vi "readRawFile.vi"() -> ()   [LabVIEW 2017]
uses:
  <vilib>/vision/NI_Vision_Development_Module.lvlib
panel:
  out "Histogram Report 2":T1 {"Standard  Variation" format="%.2f"; "Mean Value" format="%.2f"; "Interval Width" format="%.2f"; "Starting Value" format="%.2f"; "Maximal Value" format="%.2f"; "Minimal Value" format="%.2f"}
  out "Histogram Report":T1 {"Standard  Variation" format="%.2f"; "Mean Value" format="%.2f"; "Interval Width" format="%.2f"; "Starting Value" format="%.2f"; "Maximal Value" format="%.2f"; "Minimal Value" format="%.2f"}
  out "Error out":errorcluster
  in  "Raw File Path":path=path "F:/BonTechWrapperLibrary/BonTechWrapperLibrary/x64/Release/test.raw"
  in  "Length":i32=256
  in  "Frame Header":bool
  out "Image":T2(plugin-control)
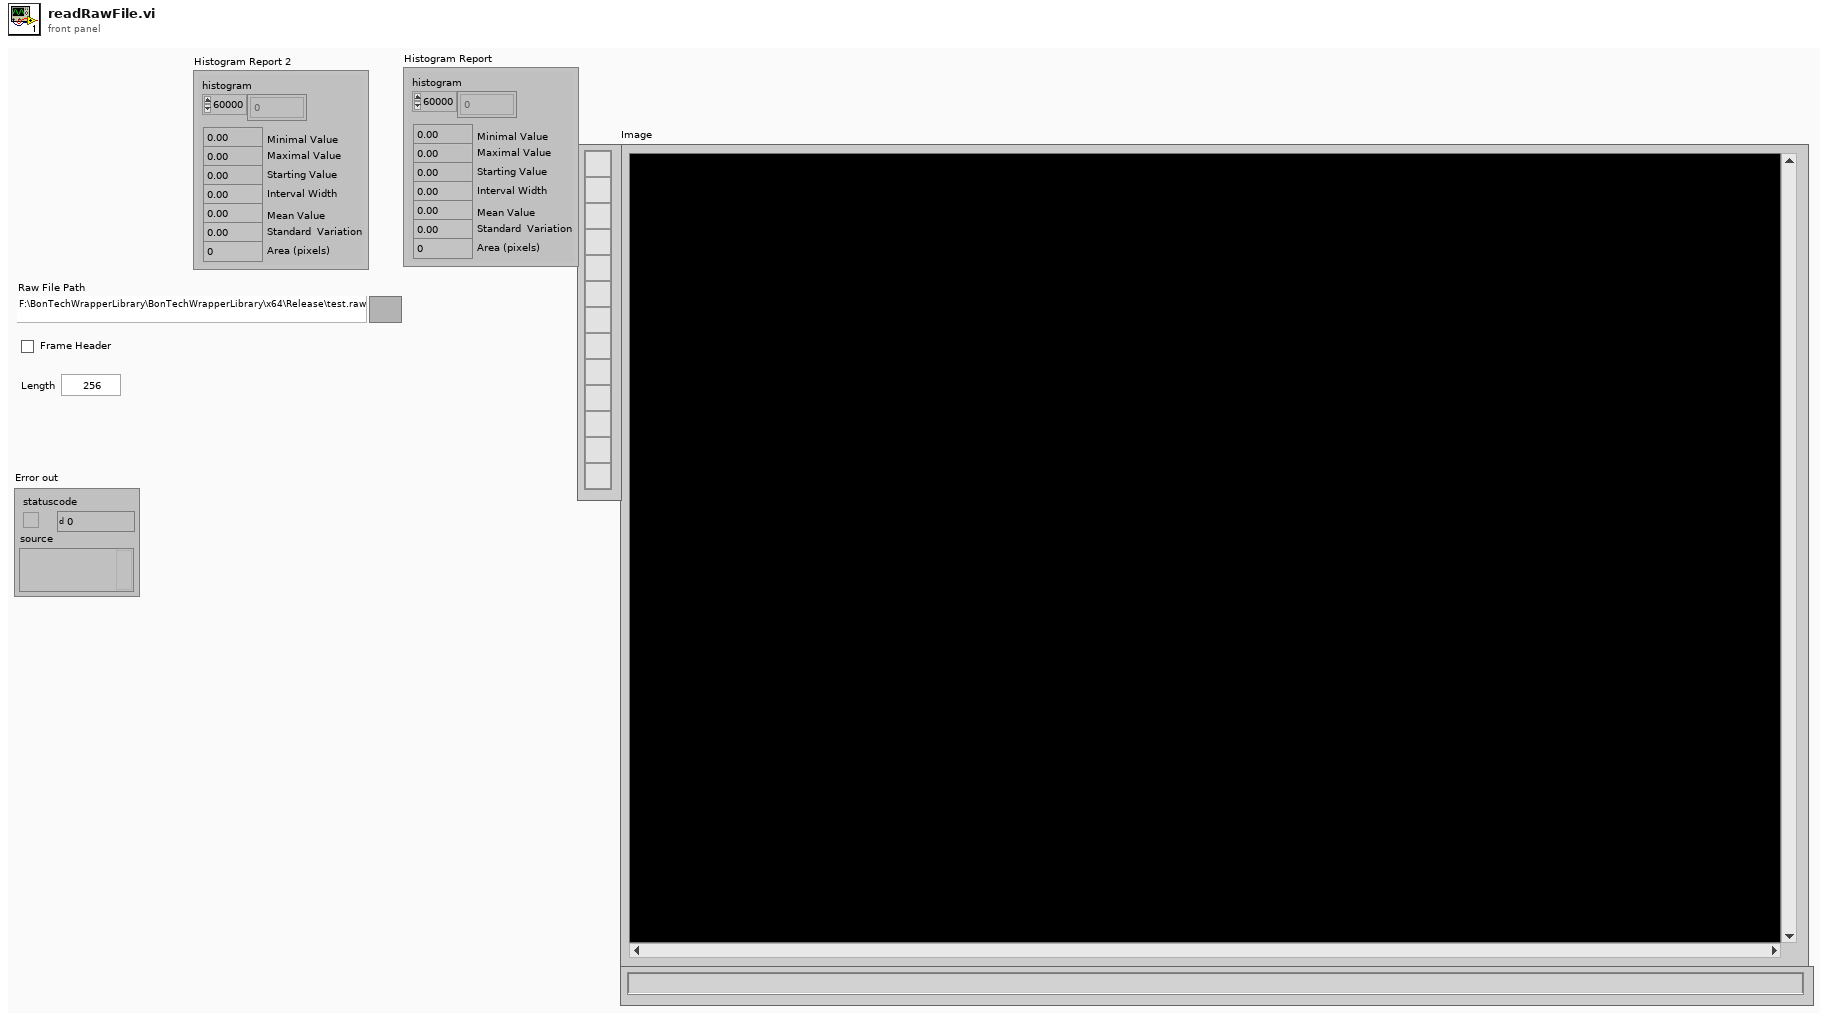
[diagram p1: front panel]
types:
  T1 = cluster{"histogram":u32[], "Minimal Value":sgl, "Maximal Value":sgl, "Starting Value":sgl, "Interval Width":sgl, "Mean Value":sgl, "Standard  Variation":sgl, "Area (pixels)":i32}
  T2 = typedef "IMAQ Image.ctl" = refnum<image>
  T3 = cluster{"Conversion Method":u32, "Minimum Value":i32, "Maximum Value":i32, "Number Of Shifts":i32}
  T4 = typedef "Image Type" = u32
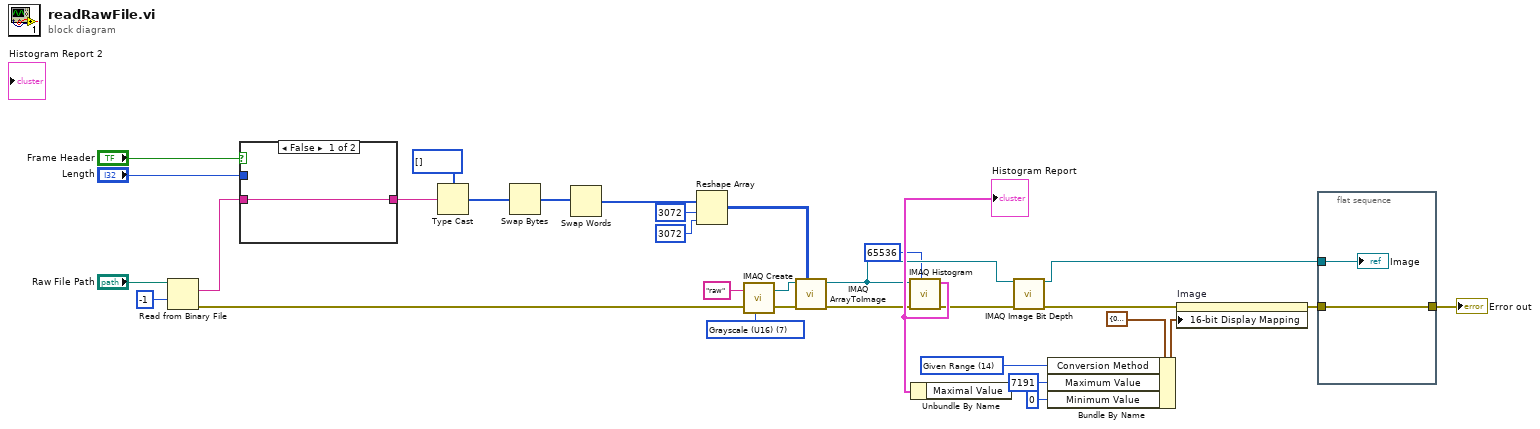
[diagram p0: block diagram]
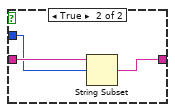
[diagram p2: hidden frame]
diagram:
  w11 = u32 14 items=["Default"=10, "Most Significant Bits"=11, "Full Dynamic"=12, "Downshift"=13, "Given Range"=14, "90% Dynamic"=15, "Given Percent Range"=16] ("16-bit Display Mapping:Conversion Method")
  w28 = T4 7 items=["Grayscale (U8)", "Grayscale (I16)", "Grayscale (SGL)", "Complex (CSG)", "RGB (U32)", "HSL (U32)", "RGB (U64)", "Grayscale (U16)"] ("Image Type")
  n1 = Read from Binary File(10:-1 ("count (1)"), 11:"Raw File Path") -> (0:w18:errorcluster, 2:w21:string)  [unwired: 4 in, 2 out]
  n2 = case shown="False" "Frame Header" {
    tunnel: w21 -> [w33 w36]
    tunnel: "Length" -> [_ w34]
    tunnel: [w33 w35] -> w19
    frame False {
    }
    frame True {
      n3 = String Subset(string=w36, offset (0)=w34) -> (substring=w35:string)  [unwired: 1 in]
    }
  }
  n4 = Type Cast(type=u16[] [], x=w19) -> (*(type *) &x=w16:u16[])
  n5 = Swap Bytes(anything=w16) -> (byte swapped=w17:u16[])
  n6 = Swap Words(1:w17) -> (0:w15:u16[])
  n7 = Reshape Array(w15, 3072 ("dimension size"), 3072 ("dimension size")) -> (w24:u16[][])
  n8 = call "IMAQ Create"("Image Name"="raw", "Image Type"=w28, "error in (no error)"=w18) -> ("New Image"=w27:T2, "error out"=w23:errorcluster)  [unwired: 2 in]
  n9 = call "IMAQ ArrayToImage"("Image Pixels (U16)"=w24, "error in (no error)"=w23, "Image"=w27) -> ("error out"=w10:errorcluster, "Image Out"=w7:T2)  [unwired: 7 in]
  n10 = call "IMAQ Histogram"("Number of Classes"=65536, "error in (no error)"=w10, "Image"=w7) -> ("error out"=w5:errorcluster, "Histogram Report"=w14:T1)  [unwired: 7 in]
  "Histogram Report" <- w14
  n11 = Unbundle By Name(w14) -> ()  [unwired: 1 out]
  n12 = call "IMAQ Image Bit Depth"("Image"=w7, "error in (no error)"=w5) -> ("Image Out"=w6:T2, "error out"=w4:errorcluster)  [unwired: 11 in, 1 out]
  n13 = Bundle By Name(cluster=T3 {"Conversion Method"=0, "Minimum Value"=0, "Maximum Value"=0, "Number Of Shifts"=0} ("16-bit Display Mapping:All Elements"), "Conversion Method"=w11, "Maximum Value"=7191, "Minimum Value"=0) -> (w12:T3)
  n14 = property on="Image" class="ImageControl"(error in=w4, "16-bit Display Mapping"=w12) -> (error out=w9:errorcluster)  [unwired: 1 in, 1 out]
  n15 = flat-sequence {
    tunnel: w9 -> [w38]
    tunnel: [w38] -> w8
    tunnel: w6 -> [w37]
    frame #0 {
      "Image" <- w37
    }
  }
  "Error out" <- w8
